vi "Calculator_Using_Event_Structure.vi"() -> ()   [LabVIEW 2017, in "Examples.lvlib"]
uses:
  Examples.lvlib
panel:
  out "?":string
  in  "Multiply":bool
  in  "=":bool
  in  "Clear":bool
  in  ".":bool
  in  "0":bool
  in  "Divide":bool
  in  "3":bool
  in  "2":bool
  in  "1":bool
  in  "Minus":bool
  in  "6":bool
  in  "5":bool
  in  "4":bool
  in  "Plus":bool
  in  "9":bool
  in  "8":bool
  in  "7":bool
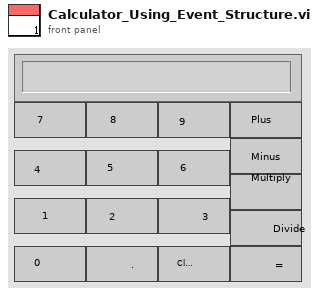
[diagram p1: front panel]
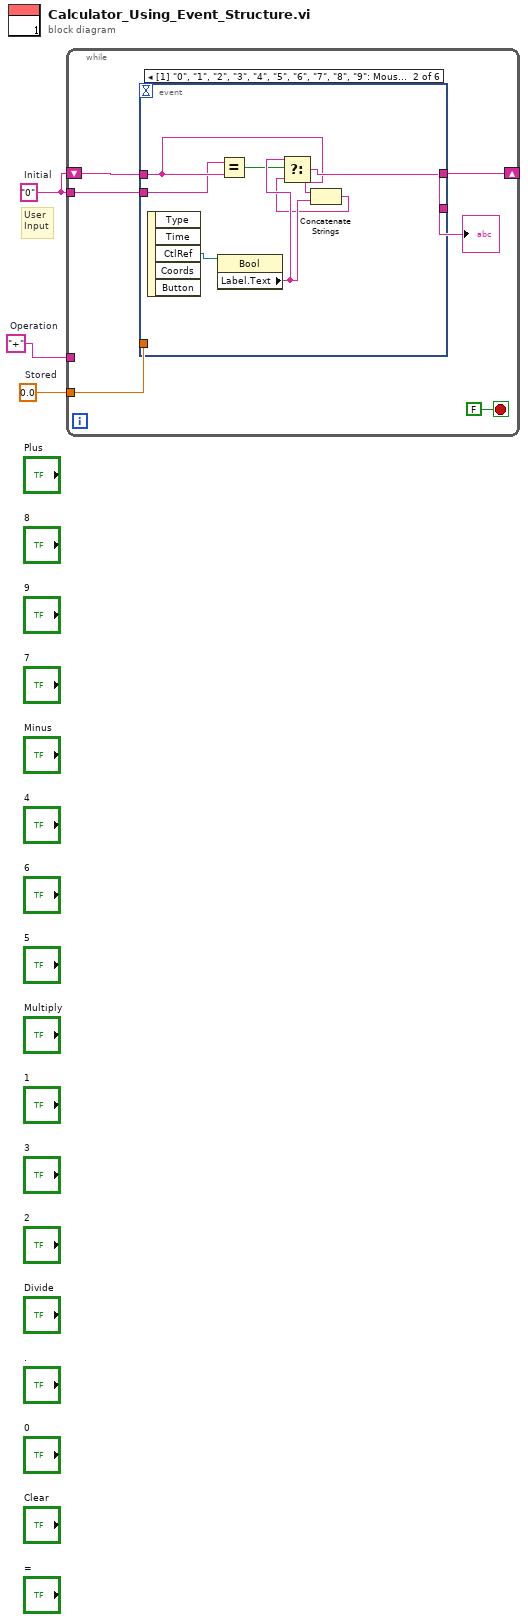
[diagram p0: block diagram]
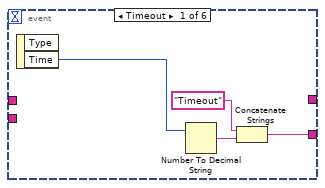
[diagram p2: hidden frame]
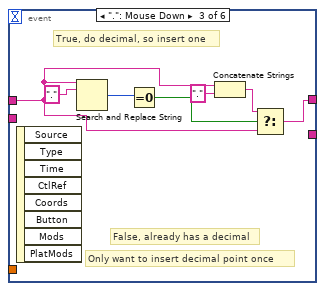
[diagram p3: hidden frame]
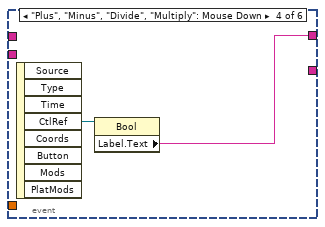
[diagram p4: hidden frame]
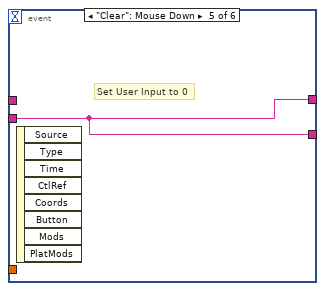
[diagram p5: hidden frame]
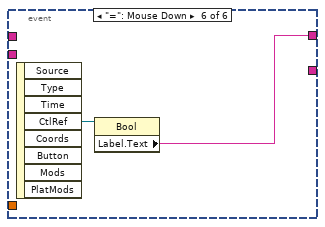
[diagram p6: hidden frame]
diagram:
  w1 = 0.0  # Stored
  w2 = "+"  # Operation
  w3 = "0"  # Initial
  # "User\nInput"
  n1 = while {
    shift-right: [w5] -> _
    shift-left: w3 -> [w8]
    tunnel: w3 -> [w6]
    tunnel: w2 -> [_]
    tunnel: w1 -> [w4]
    stop <- FALSE stop-if-true
    n2 = event shown="[1] \"0\", \"1\", \"2\", \"3\", \"4\", \"5\", \"6\", \"7\", \"8\", \"9\": Mouse Down" {
      selector: _ -> [_ _ _ _ _ _]
      dyn-events: _ -> [_ _ _ _ _ _]
      timeout: _ -> [_ _ _ _ _ _]
      tunnel: [w9 _ _ _ w29 _] -> _
      tunnel: w8 -> [_ w15 w22 _ _ _]
      tunnel: [_ w16 w23 w27 w29 w30] -> w5
      tunnel: w6 -> [_ w14 _ _ w29 _]
      tunnel: w4 -> [_ _ _ _ _ _]
      event Timeout {
        n3 = event-data() -> ("Time"=w12:u32)  [unwired: 1 in, 1 out]
        n4 = Number To Decimal String(number=w12) -> (decimal integer string=w11:string)  [unwired: 1 in]
        n5 = Concatenate Strings("Timeout", w11) -> (w9:string)
      }
      event "0", "1", "2", "3", "4", "5", "6", "7", "8", "9": Mouse Down {
        n6 = event-data() -> ("CtlRef"=w19:refnum<vi>)  [unwired: 1 in, 4 out]
        n7 = property class="Bool"(reference=w19) -> ("Label.Text"=w18:string)  [unwired: 1 in, 2 out]
        n8 = Equal?(x=w14, y=w15) -> (x = y?=w13:bool)
        n9 = Concatenate Strings(w15, w18) -> (w17:string)
        n10 = Select(t=w18, s=w13, f=w17) -> (s? t:f=w16:string)
      }
      event ".": Mouse Down {
        # "False, already has a decimal"
        # "True, do decimal, so insert one"
        # "Only want to insert decimal point once"
        n11 = event-data() -> ()  [unwired: 1 in, 8 out]
        n12 = Search and Replace String(input string=w22, search string="." ("input string")) -> (number of replacements=w25:i32)  [unwired: 6 in, 3 out]
        n13 = Equal To 0?(x=w25) -> (x = 0?=w24:bool)
        n14 = Concatenate Strings(w22, "." ("string")) -> (w20:string)
        n15 = Select(t=w20, s=w24, f=w22) -> (s? t:f=w23:string)
      }
      event "Plus", "Minus", "Divide", "Multiply": Mouse Down {
        n16 = event-data() -> ("CtlRef"=w28:refnum<vi>)  [unwired: 1 in, 7 out]
        n17 = property class="Bool"(reference=w28) -> ("Label.Text"=w27:string)  [unwired: 1 in, 2 out]
      }
      event "Clear": Mouse Down {
        # "Set User Input to 0"
        n18 = event-data() -> ()  [unwired: 1 in, 8 out]
      }
      event "=": Mouse Down {
        n19 = event-data() -> ("CtlRef"=w31:refnum<vi>)  [unwired: 1 in, 7 out]
        n20 = property class="Bool"(reference=w31) -> ("Label.Text"=w30:string)  [unwired: 1 in, 2 out]
      }
    }
    "?" <- w5
  }
